vi "Update-acquire-timeout.vi"(8 "error in":errorcluster, 10 "UI ref. in":refnum<data-value>, 11 "Data ref. in":refnum<data-value>) -> (0 "error IO":errorcluster, 2 "UI ref.":refnum<data-value>, 3 "Data ref.":refnum<data-value>)   [LabVIEW 2013, in "CameraVision.lvlib" / "CV-Main.lvclass"]
doc: "This function sets the time at which the acquisition is stopped automatically, based on the current time and the user specified 'Max. duration'.\n\nThe image acquisition can be stopped sooner by using the 'Stop' button, by closing the program window or by choosing 'Single batch' as the acquisition mode, with a low batch size.\n\nThis setting is also active for a virtual acquisition (using imported images)."
uses:
  CV-Main.lvclass
  UI/CV-UI.lvclass
  UI/CV-UI.lvclass/CV-UI.ctl
  CV-Main.lvclass/CV-Main.ctl
  Acquisition/CV-Acquisition.lvclass/CV-Acquisition.ctl
  Acquisition/Read Duration HH.vi
  Acquisition/Read Duration MM.vi
  Acquisition/Read Duration SS.vi
  Read Acquis params.vi
  UI/Read Acquire stop.vi
  Acquisition/CV-Acquisition.lvclass
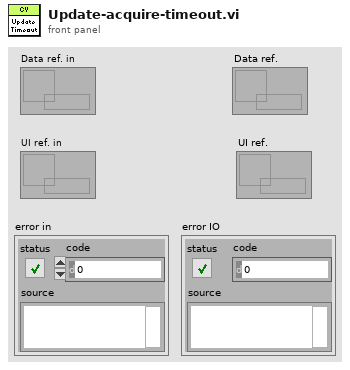
[diagram p1: front panel]
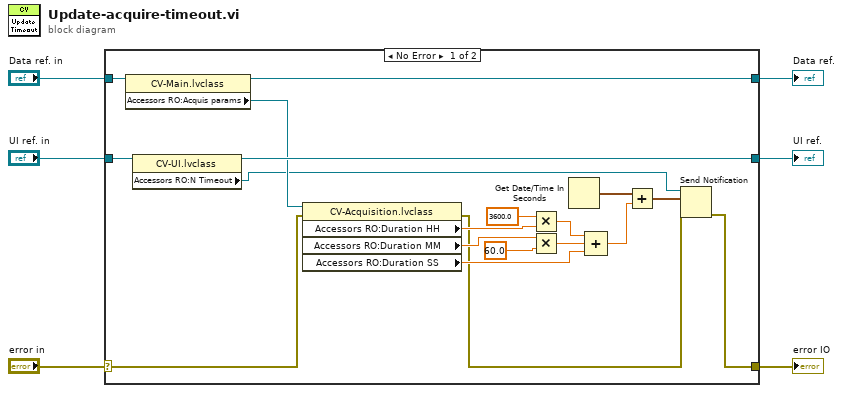
[diagram p0: block diagram]
diagram:
  n1 = case shown="No Error" "error in" {
    selector: "error in" -> [w14 w28]
    tunnel: [w18 w28] -> w6
    tunnel: "Data ref. in" -> [w12 w26]
    tunnel: [w11 w26] -> w3
    tunnel: "UI ref. in" -> [w10 w27]
    tunnel: [w9 w27] -> w1
    frame No Error {
      n2 = property class="CV-Main.lvclass"(reference=w12) -> (reference out=w11:refnum<data-value>, "Accessors RO:Acquis params"=w8:refnum<data-value>)  [unwired: 1 in, 1 out]
      n3 = property class="CV-UI.lvclass"(reference=w10) -> (reference out=w9:refnum<data-value>, "Accessors RO:N Timeout"=w7:refnum<notifier>)  [unwired: 1 in, 1 out]
      n4 = property class="CV-Acquisition.lvclass"(reference=w8, error in=w14) -> (error out=w13:errorcluster, "Accessors RO:Duration HH"=w17:sgl, "Accessors RO:Duration MM"=w16:sgl, "Accessors RO:Duration SS"=w15:sgl)  [unwired: 1 out]
      n5 = Multiply(x=sgl 3600.0, y=w17) -> (x*y=w22:sgl)
      n6 = Multiply(x=w16, y=sgl 60.0) -> (x*y=w21:sgl)
      n7 = Get Date/Time In Seconds() -> (seconds since 1Jan1904=w24:timestamp)
      n8 = Compound Arithmetic op=ADD(w22, w21, w15) -> (w23:sgl)
      n9 = Add(x=w24, y=w23) -> (x+y=w25:timestamp)
      n10 = Send Notification(notification=w25, notifier=w7, error in (no error)=w13) -> (error out=w18:errorcluster)  [unwired: 1 out]
    }
    frame Error {
    }
  }
  "error IO" <- w6
  "Data ref." <- w3
  "UI ref." <- w1
